vi "GetControlUID.vi"(6 "error in":errorcluster, 9 "Control Terminal in":refnum<class "ControlTerminal.lvclass">) -> (0 "error out":errorcluster, 3 "Control Terminal out":refnum<class "ControlTerminal.lvclass">, 4 "control UID":i32)   [LabVIEW 2014, in "ControlTerminal.lvclass"]
uses:
  ControlTerminal.lvclass
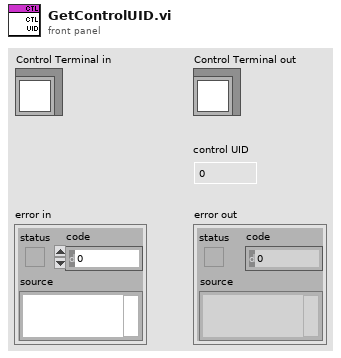
[diagram p1: front panel]
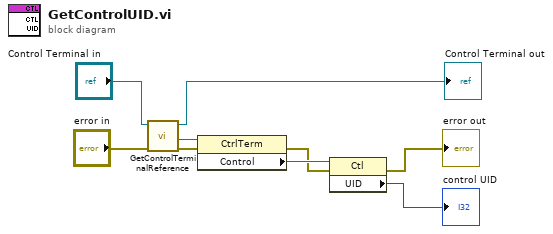
[diagram p0: block diagram]
diagram:
  n1 = call "GetControlTerminalReference.vi"("error in"="error in", "ControlTerminal in"="Control Terminal in") -> ("error out"=w5:errorcluster, "reference"=w4:refnum<vi>, "ControlTerminal out"=→"Control Terminal out":refnum<class "ControlTerminal.lvclass">)  [unwired: 7 in]
  n2 = property class="CtrlTerm"(reference=w4, error in=w5) -> (error out=w8:errorcluster, "Control"=w9:refnum<vi>)  [unwired: 1 out]
  n3 = property class="Ctl"(reference=w9, error in=w8) -> (error out=→"error out":errorcluster, "UID"=→"control UID":i32)  [unwired: 1 out]
